vi "ErrorHandler.vi"(0 "[error code] (0)":i32 format="%0.0f", 1 "[error source] (\" \")":string, 3 "type of dialog (OK msg:1)":T2=1 items=["no dialog", "OK message", "continue or stop message", "OK message + warnings", "continue/stop + warnings"], 5 "error in (no error)":errorcluster, 7 "[exception action] (none:0)":i32(ring) items=["no exception", "cancel error on match", "set error on match"], 9 "[exception code]":i32 format="%0.0f", 11 "[exception source]":string) -> (13 "HGF_Severity":T1=enum."Error", 14 "error?":bool, 15 "code out":i32 format="%0.0f", 16 "source out":string, 17 "message":string=" INSTRUCTIONS:\r\rNormal Use:  When using subVIs that incorporate the error in/error out (or error I/O) structure, place this handler where you want to inform the user of an error, typically at the end of the I/O data path, as the last action of the program.  If the error in error? is ERROR, the handler creates a message describing the error and its source.  If the type of dialog = 1 (default), the message is displayed to the user, who can only acknowedge it.  If the type = 2, the user can acknowledge the message or abort execution; aborting a program with active I/O is not recommended.  If the type = 0, no message is displayed; this is used to process the error programmatically, and the error out cluster elements are wired to individual terminals for that reason.  \r\rOther Use:\n\r\nlocal testing.  To test the error code of a subVI or function that does not have the error I/O structure, you can wire its error code and a source string to the local error code and error source inputs.  If error in error? indicates no error and error code is not equal to 0, the local code and source are substituted for the error in values, and error? is set TRUE (ERROR).", 19 "error out":errorcluster)   [LabVIEW 2012, in "HGF_Auxiliary.lvlib"]
doc: "Indicates whether an error occurred. If an error occurred, this VI returns a description of the error and severity and optionally displays a dialog box."
uses:
  HGF_Auxiliary.lvlib
  <vilib>/Utility/error.llb/DialogType.ctl
  Severity.ctl
  ErrorCode.ctl
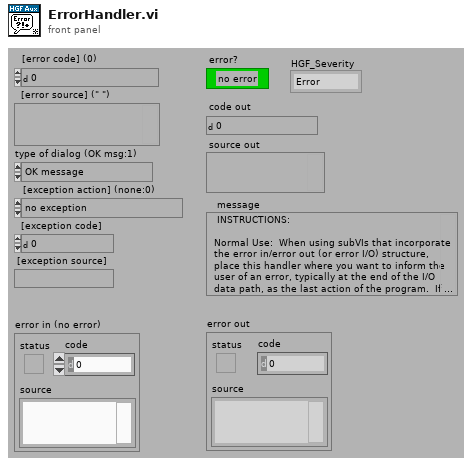
[diagram p1: front panel]
types:
  T1 = typedef "HGF_Auxiliary.lvlib/Severity.ctl" = enum16{"Info", "Warning", "Fault", "Error", "Fatal"}
  T2 = typedef "DialogType.ctl" = u16
  T3 = typedef "HGF_Auxiliary.lvlib/ErrorCode.ctl" = enum32{"No error", "Function not supported.", "This VI is for friends only.", "Reference object aready exisits.", "Parameter out of range.", "Not a rendezvous.", "Invalid notifier reference.", "Invalid queue reference.", "Self-Test not supported.", "Reset not supported.", "IDN query not supported.", "Error query not supported.", "Incorrect addressee.", "Object already exists.", "No class name specified", "Driver not supported", "Attribute is not writable"}
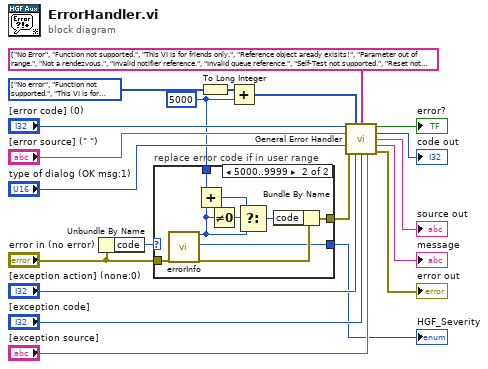
[diagram p0: block diagram]
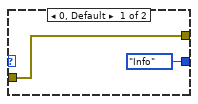
[diagram p2: hidden frame]
diagram:
  w5 = 5000
  w8 = T3[] [enum."No error", enum."Function not supported.", enum."This VI is for friends only.", enum."Reference object aready exisits.", enum."Parameter out of range.", enum."Not a rendezvous.", enum."Invalid notifier reference.", enum."Invalid queue reference.", enum."Self-Test not supported.", enum."Reset not supported.", enum."IDN query not supported.", enum."Error query not supported.", enum."Incorrect addressee.", enum."Object already exists.", enum."No class name specified", enum."Attribute is not writable"] items=["No error", "Function not supported.", "This VI is for friends only.", "Reference object aready exisits.", "Parameter out of range.", "Not a rendezvous.", "Invalid notifier reference.", "Invalid queue reference.", "Self-Test not supported.", "Reset not supported.", "IDN query not supported.", "Error query not supported.", "Incorrect addressee.", "Object already exists.", "No class name specified", "Driver not supported", "Attribute is not writable"] ("[user-defined codes]")
  n1 = Unbundle By Name("error in (no error)") -> ("code"=w1:i32)
  n2 = case "replace error code if in user range" shown="5000..9999" w1 {
    tunnel: w5 -> [_ w31]
    tunnel: "error in (no error)" -> [w22 w30]
    tunnel: [Severity."Info" ("HGF_Severity") w28] -> w4
    tunnel: [w22 w27] -> w3
    frame 0, Default {
    }
    frame 5000..9999 {
      n3 = call "errorInfo.vi"("error in (no error)"=w30) -> ("HGF_Error"=w23:T3, "HGF_Severity"=w28:T1, "error out"=w29:errorcluster)  [unwired: 16 out]
      n4 = Add(x=w31, y=w23) -> (x+y=w26:u32)
      n5 = Not Equal To 0?(x=w23) -> (x != 0?=w24:bool)
      n6 = Select(t=w26, s=w24, f=w23) -> (s? t:f=w25:u32)
      n7 = Bundle By Name(cluster=w29, "code"=w25) -> (w27:errorcluster)
    }
  }
  "HGF_Severity" <- w4
  n8 = To Long Integer(number=w8) -> (32bit integer=w7:i32[])
  n9 = Add(x=w7, y=w5) -> (x+y=w6:i32[])
  n10 = call <vilib>:"General Error Handler.vi"("[error code] (0)"="[error code] (0)", "[user-defined codes]"=w6, "[user-defined descriptions]"=string[] ["No Error", "Function not supported.", "This VI is for friends only.", "Reference object aready exisits!", "Parameter out of range.", "Not a rendezvous.", "Invalid notifier reference.", "Invalid queue reference.", "Self-Test not supported.", "Reset not supported.", "IDN query not supported.", "Error query not supported.", "Incorrect addressee.", "Object already exists.", "No class name specified.", "Attribute is not writable."], "[error source] (\" \")"="[error source] (\" \")", "type of dialog (OK msg:1)"="type of dialog (OK msg:1)", "error in (no error)"=w3, "[exception action] (none:0)"="[exception action] (none:0)", "[exception code]"="[exception code]", "[exception source]"="[exception source]") -> ("error?"=→"error?":bool, "code out"=→"code out":i32, "source out"=→"source out":string, "message"=→"message":string, "error out"=→"error out":errorcluster)  [unwired: 2 out]
